vi "Suspend.vi"(8 "error in (no error)":errorcluster, 11 "Motor-Maxon in":refnum<class "Motor-Maxon.lvclass">) -> (0 "error out":errorcluster, 3 "Motor-Maxon out":refnum<class "Motor-Maxon.lvclass">)   [LabVIEW 2013, in "PowderDeposition.lvlib" / "Motor-Maxon.lvclass"]
uses:
  Motor-Maxon.lvclass
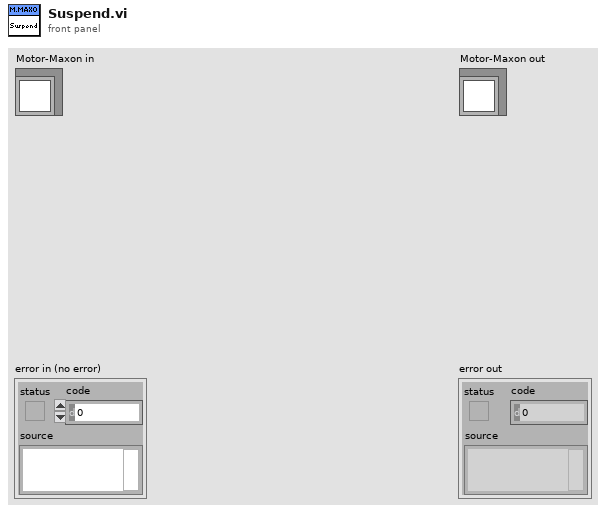
[diagram p1: front panel]
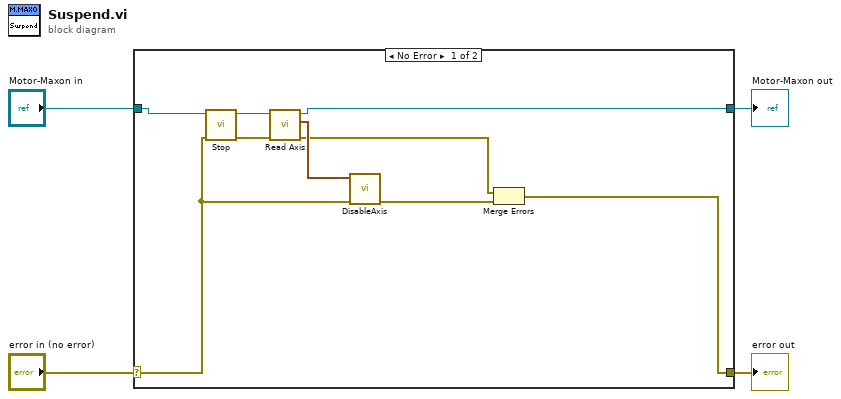
[diagram p0: block diagram]
diagram:
  n1 = case shown="No Error" "error in (no error)" {
    selector: "error in (no error)" -> [w7 w15]
    tunnel: [w6 w15] -> w3
    tunnel: [w8 w14] -> w1
    tunnel: "Motor-Maxon in" -> [w13 w14]
    frame No Error {
      n2 = call-dynamic "Stop.vi"("error in (no error)"=w7, "Motor-Maxon in"=w13) -> ("error out"=w10:errorcluster, "Motor-Maxon out"=w12:refnum<class "Motor-Maxon.lvclass">)  [unwired: 8 in]
      n3 = call-dynamic "Read Axis.vi"("error in (no error)"=w10, "Motor-Maxon in"=w12) -> ("error out"=w9:errorcluster, "Axis"=w11:cluster{"keyHandle":u32, "nodeID":u16}, "Motor-Maxon out"=w8:refnum<class "Motor-Maxon.lvclass">)  [unwired: 7 in]
      n4 = call <instrlib>:"DisableAxis.vi"("error in (no error)"=w7, "axis in"=w11) -> ("error out"=w5:errorcluster)  [unwired: 4 in, 1 out]
      n5 = Merge Errors(w9, w5) -> (w6:errorcluster)
    }
    frame Error {
    }
  }
  "error out" <- w3
  "Motor-Maxon out" <- w1
